vi "Nattify - Arrange FP.vi"(0 "VI in":refnum<vi>, 11 "error in":errorcluster) -> (4 "VI out":refnum<vi>, 15 "error out":errorcluster)   [LabVIEW 2020]
uses:
  <vilib>/Utility/traverseref.llb/TRef TravTarget.ctl
  Nattify - Window Type.ctl
  <vilib>/Utility/miscctls.llb/LVPointTypeDef.ctl
  <vilib>/Utility/traverseref.llb/VI Scripting - Traverse.lvlib
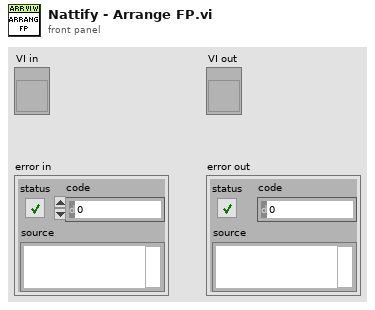
[diagram p1: front panel]
types:
  T1 = typedef "TRef TravTarget.ctl" = enum16{"FP", "BD", "Other"}
  T2 = typedef "Nattify - Window Type.ctl" = enum16{"FP", "BD"}
  T3 = typedef "LVPointTypeDef.ctl" = cluster{"Horizontal":i16, "Vertical":i16}
  T4 = typedef "LVRectTypeDef.ctl" = cluster{"Left":i16, "Top":i16, "Right":i16, "Bottom":i16}
  T5 = typedef "Nattify - Min Window Dimensions.ctl" = cluster{"min window width":i16, "min window height":i16}
  T6 = typedef "Nattify - Window Gaps.ctl" = cluster{"left gap":i16, "top gap":i16, "min right gap":i16, "min bottom gap":i16}
  T7 = cluster{"display workspace bounds":T4, "min window dimensions":T5, "window gaps":T6}
  T8 = typedef "Nattify - FP Objects Arrangement Info.ctl" = cluster{"grid size":i32, "horizontal margin factor":i32, "horizontal spacing factor":i32, "vertical margin factor":i32, "vertical spacing factor":i32}
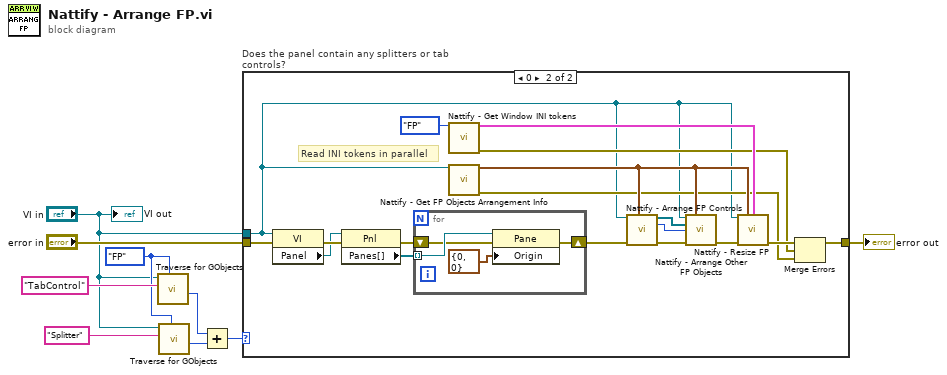
[diagram p0: block diagram]
diagram:
  w6 = TRef_TravTarget."FP" ("Traverse Target")
  n1 = call <vilib>:"Traverse for GObjects.vi"("Traverse Target"=w6, "Class Name"="TabControl", "VI Refnum"="VI in") -> ("# of Refs"=w4:i32)  [unwired: 5 in, 3 out]
  n2 = call <vilib>:"Traverse for GObjects.vi"("Traverse Target"=w6, "Class Name"="Splitter", "VI Refnum"="VI in") -> ("# of Refs"=w3:i32)  [unwired: 5 in, 3 out]
  n3 = Add(x=w4, y=w3) -> (x+y=w2:i32)
  n4 = case "Does the panel contain any splitters or tab controls?" shown="0" w2 {
    tunnel: "error in" -> [w10 w19]
    tunnel: [w10 w14] -> w8
    tunnel: "VI in" -> [_ w11]
    frame Default {
      # "Plugin will no-op on a panel with a splitter or tab control."
    }
    frame 0 {
      # "Read INI tokens in parallel"
      n5 = property class="VI"(reference=w11, error in=w19) -> (error out=w25:errorcluster, "Panel"=w24:refnum<vi>)  [unwired: 1 out]
      n6 = property class="Pnl"(reference=w24, error in=w25) -> (error out=w26:errorcluster, "Panes[]"=w27:refnum<vi>[])  [unwired: 1 out]
      n7 = for {
        tunnel: w27 -> [w32] mode=indexing
        shift-right: [w30] -> w17
        shift-left: w26 -> [w31]
        n8 = property class="Pane"(reference=w32, error in=w31, "Origin"=T3 {"Horizontal"=0, "Vertical"=0}) -> (error out=w30:errorcluster)  [unwired: 1 out]
      }
      n9 = call "Nattify - Get Window INI tokens.vi"("window type"=Nattify_-_Window_Type."FP") -> ("Window INI tokens"=w16:T7, "error out"=w13:errorcluster)  [unwired: 13 in]
      n10 = call "Nattify - Get FP Objects Arrangement Info.vi"("VI reference"=w11) -> ("FP objects arrangement info"=w20:T8, "error out"=w12:errorcluster)  [unwired: 13 in]
      n11 = call "Nattify - Arrange FP Controls.vi"("VI in"=w11, "FP objects arrangement info"=w20, "error in"=w17) -> ("controls from conn pane"=w22:refnum<vi>[], "max bottom"=w21:i16, "error out"=w28:errorcluster)  [unwired: 10 in]
      n12 = call "Nattify - Arrange Other FP Objects.vi"("VI in"=w11, "FP objects arrangement info"=w20, "controls from conn pane"=w22, "max bottom of arranged controls"=w21, "error in"=w28) -> ("error out"=w23:errorcluster)  [unwired: 10 in]
      n13 = call "Nattify - Resize FP.vi"("VI in"=w11, "FP objects arrangement info"=w20, "Window INI tokens"=w16, "error in"=w23) -> ("error out"=w18:errorcluster)  [unwired: 11 in]
      n14 = Merge Errors(w18, w13, w12) -> (w14:errorcluster)
    }
  }
  "error out" <- w8
  "VI out" <- "VI in"
